vi "Keithley 6517A V-Source Outp.vi"(1 "Vsource Voltage Limit":dbl min=0.0 max=1000.0 step=0.005 format="%.3f", 2 "Output Voltage Value":dbl min=0.0 max=1000.0 step=0.005 format="%.3f", 3 "V-Source Range (100:0)":u16(ring) items=["+/- 100 Volts", "+/- 1000 Volts"], 4 "Resistive Current Limit":bool, 5 "Voltage Limit State":bool, 6 "V-Source Operate":bool, 8 "error in":T1, 10 "Vsource Control Selection":u16(ring) items=["Set Vsource Output On/Off State", "Set Vsource Range and Output Level", "Set Vsource Voltage Limit and State", "Enable Measure Connect", "Disable Measure Connect", "Set Resistive Current Limit State"], 11 "GPIB address":string="27") -> (0 "error out":T1)   [LabVIEW 2015]
doc: "This VI is used to set the Built-In Voltage Source. The user can select either a +/- 100 Volt range or a +/- 1000 Volt range. The desired output can be selected and the output can be turned on or off. Note that if the range is set for +/- 100 V and the selected output voltage is greater than 100 volts, the output will clamp at 100 volts. To get a voltage higher than 100, you must select the +/-1000 volt range.\n\nParameters:\nVsource Control Selection:\n0 = Set Vsource Output On/Off State\n1 = Set Vsource Range and Output Level\n2 = Set Vsource Voltage Limit and State\n3 = Enable Measure Connect\n4 = Disable Measure Connect\n5 = Set Resistive Current Limit State\n\nV-source Operate:\nTRUE = Operate\nFALSE = Standby\n\nResistive Current Limit\nTRUE = Operate\nFALSE = Standby\n\nVoltage Limit State:\nTRUE = Operate\nFALSE = Standby"
panel:
  # "Operate\nStandby"
  # "On\nOff"
  # "Enabled\nDisabled"
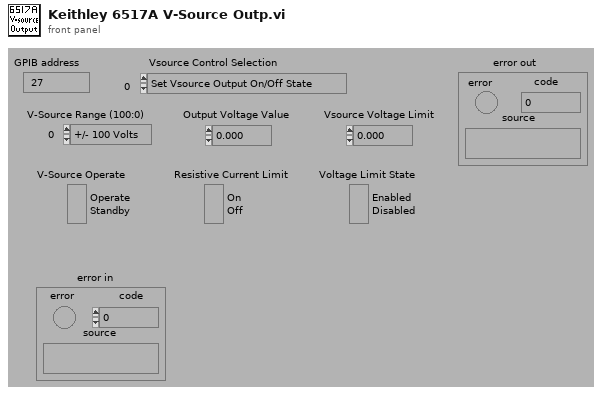
[diagram p1: front panel]
types:
  T1 = cluster{"error":bool, "code":i32, "source":string}
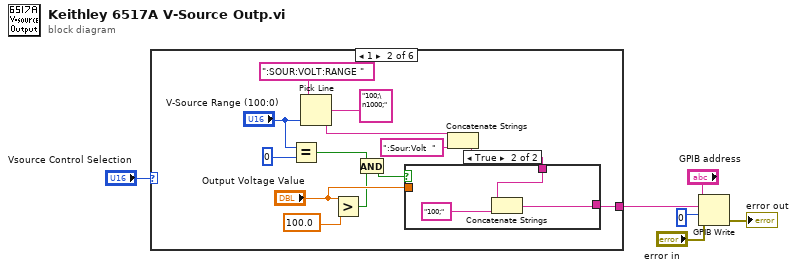
[diagram p0: block diagram]
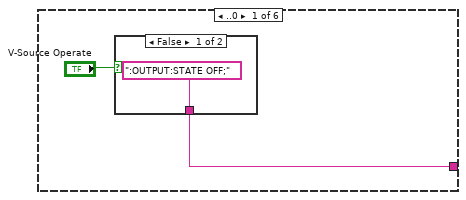
[diagram p2: hidden frame]
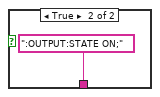
[diagram p3: hidden frame]
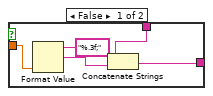
[diagram p4: hidden frame]
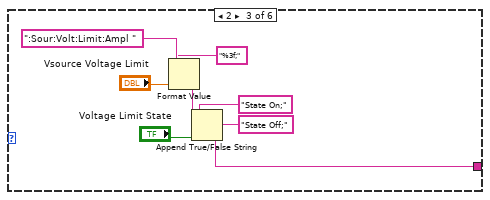
[diagram p5: hidden frame]
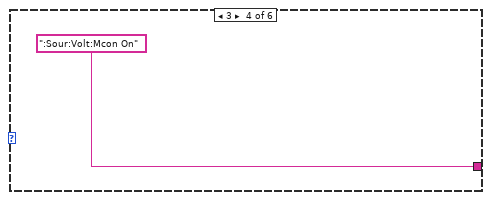
[diagram p6: hidden frame]
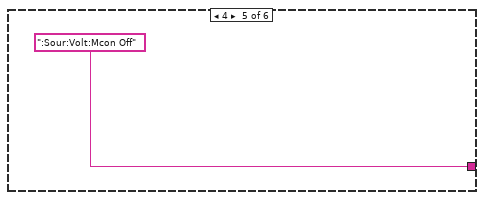
[diagram p7: hidden frame]
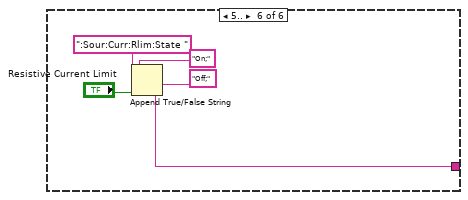
[diagram p8: hidden frame]
diagram:
  n1 = case shown="1" "Vsource Control Selection" {
    tunnel: [w7 w11 w32 ":Sour:Volt:Mcon On" ":Sour:Volt:Mcon Off" w42] -> w1
    frame ..0 {
      n2 = case shown="False" "V-Source Operate" {
        tunnel: [":OUTPUT:STATE OFF;" ":OUTPUT:STATE ON;"] -> w7
        frame False {
        }
        frame True {
        }
      }
    }
    frame 1 {
      n3 = Equal?(x="V-Source Range (100:0)", y=0) -> (x = y?=w17:bool)
      n4 = Pick Line(string ("")=":SOUR:VOLT:RANGE ", multi-line string="100;\n1000;", line index="V-Source Range (100:0)") -> (output string=w20:string)
      n5 = Greater?(x="Output Voltage Value", y=sgl 100.0) -> (0:w18:bool)
      n6 = And(x=w17, y=w18) -> (x .and. y?=w19:bool)
      n7 = Concatenate Strings(w20, ":Sour:Volt  ") -> (w23:string)
      n8 = case shown="True" w19 {
        tunnel: "Output Voltage Value" -> [w27 _]
        tunnel: [w28 w30] -> w11
        tunnel: w23 -> [w24 w29]
        frame False {
          n9 = Format Value(format string="%.3f;", value (0)=w27) -> (output string=w25:string)  [unwired: 1 in]
          n10 = Concatenate Strings(w24, w25) -> (w28:string)
        }
        frame True {
          n11 = Concatenate Strings(w29, "100;") -> (w30:string)
        }
      }
    }
    frame 2 {
      n12 = Format Value(string ("")=":Sour:Volt:Limit:Ampl ", format string="%3f;", value (0)="Vsource Voltage Limit") -> (output string=w35:string)
      n13 = Append True/False String(1:"Voltage Limit State", 2:"State Off;", 3:"State On;", 4:w35) -> (0:w32:string)
    }
    frame 3 {
    }
    frame 4 {
    }
    frame 5.. {
      n14 = Append True/False String(1:"Resistive Current Limit", 2:"Off;", 3:"On;", 4:":Sour:Curr:Rlim:State ") -> (0:w42:string)
    }
  }
  n15 = GPIB Write(0:"GPIB address", 1:w1, 2:0, 3:"error in") -> (6:→"error out":errorcluster)  [unwired: 1 in, 1 out]
